vi "Get StateName.vi"(8 "error in (no error)":errorcluster, 11 "SMO":refnum<class "SMO.lvclass">) -> (0 "error out":errorcluster, 2 "StateName":string, 3 "SMO out":refnum<class "SMO.lvclass">)   [LabVIEW 2019, in "Instrument Attributes.lvlib"]
uses:
  <vilib>/JKI/JKI SMO/SMO/SMO.lvclass
  Attribute.Instrument/Attribute.Instrument.lvclass/Attribute.Instrument.ctl
  Instrument Attributes.lvlib
  SMO.Mediator/SMO.Mediator.lvclass
  Attribute.Instrument/Attribute.Instrument.lvclass
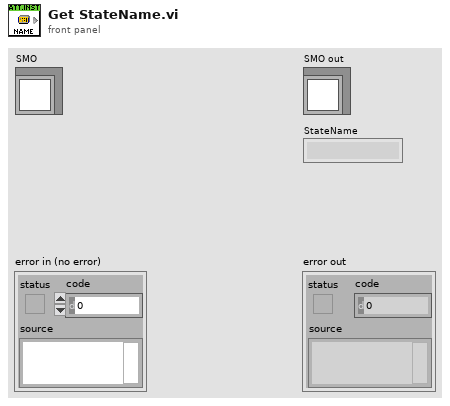
[diagram p1: front panel]
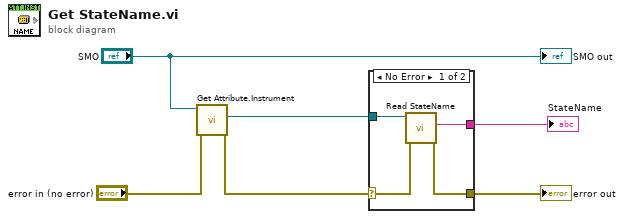
[diagram p0: block diagram]
diagram:
  n1 = call "Get Attribute.Instrument.vi"("error in (no error)"="error in (no error)", "SMO"="SMO") -> ("error out"=w3:errorcluster, "Attribute.Debug"=w4:refnum<class "Attribute.Instrument.lvclass">)  [unwired: 7 in, 1 out]
  n2 = case shown="No Error" w3 {
    selector: w3 -> [w10 _]
    tunnel: w4 -> [w8 _]
    tunnel: [w9 _] -> w2
    tunnel: [w7 _] -> w1
    frame No Error {
      n3 = call "Read StateName.vi"("error in (no error)"=w10, "Attribute.Instrument  in"=w8) -> ("error out"=w9:errorcluster, "StateName"=w7:string)  [unwired: 7 in, 1 out]
    }
    frame Error {
    }
  }
  "error out" <- w2
  "StateName" <- w1
  "SMO out" <- "SMO"
